vi "ma_SML Auto Restart One Shot Linear Weighting.vi"(0 "x(n)":dbl[](array[numeric]) format="%.2f", 1 "y(n-1)":dbl[](array[numeric]) format="%.2f", 2 "averaged sofar(n-1)":dbl, 3 "average size":dbl format="%.2f", 4 "reset?":bool) -> (5 "y(n)":dbl[](array[numeric]) format="%.2f", 6 "averaged sofar(n)":dbl, 7 "data ready?":bool)   [LabVIEW 2020, in "NI_MAPro.lvlib"]
uses:
  NI_MAPro.lvlib
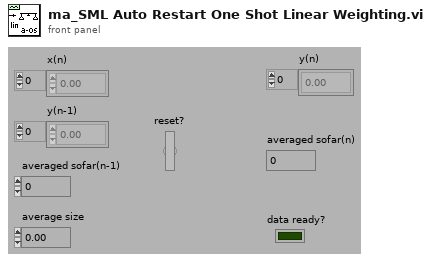
[diagram p1: front panel]
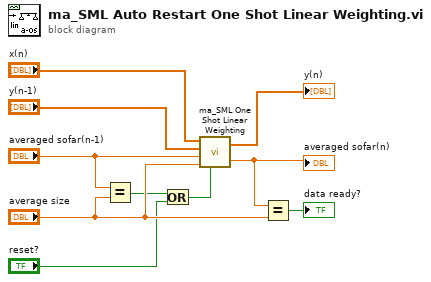
[diagram p0: block diagram]
diagram:
  n1 = Equal?(x="averaged sofar(n-1)", y="average size") -> (x = y?=w4:bool)
  n2 = Or(x=w4, y="reset?") -> (x .or. y?=w7:bool)
  n3 = call "ma_SML One Shot Linear Weighting.vi"("x(n)"="x(n)", "y(n-1)"="y(n-1)", "averaged sofar(n-1)"="averaged sofar(n-1)", "average size"="average size", "reset?"=w7) -> ("y(n)"=→"y(n)":dbl[], "averaged sofar(n)"=w1:dbl)
  "averaged sofar(n)" <- w1
  n4 = Equal?(x=w1, y="average size") -> (x = y?=→"data ready?":bool)
